vi "ROI entry-Index Zplane position.vi"(8 "error in (no error)":errorcluster, 11 "Init?":bool) -> (0 "error out":errorcluster, 3 "Z-plane selector (index)":i32)   [LabVIEW 2013]
uses:
  ROI Entry screen/Globals/gl_ROI Entry UI globals.vi
panel:
  out "Zplane position":dbl
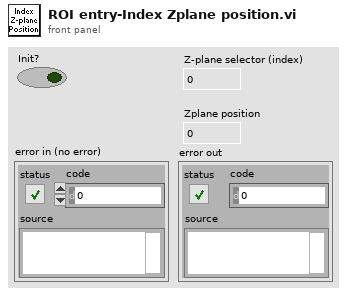
[diagram p1: front panel]
types:
  T1 = typedef "ROI entry screen ctrl refs cluster.ctl" = cluster{"Done button":refnum<vi>, "Imaging button":refnum<vi>, "Acquisition button":refnum<vi>, "POI dwell time (us)":refnum<vi>, "Scan dwell time per pixel (us)":refnum<vi>, "# of planes":refnum<vi>, "Zoom":refnum<vi>, "Equal size":refnum<vi>, "Channel":refnum<vi>, "Image Display":refnum<vi>, "Z-Plane Selector":refnum<vi>, "Number of lines left":refnum<vi>, "Z-stack folder path":refnum<vi>, "POI Density":refnum<vi>, "Arb Plane Entry":refnum<vi>, "Whole plane":refnum<vi>, "Clear Last":refnum<vi>, "Clear All":refnum<vi>, "Trial Length (sec)":refnum<vi>, "Palette Type":refnum<vi>, "Intensity slider":refnum<vi>, "# POI":refnum<vi>, "Max Z Proj":refnum<vi>, "Zplane ind":refnum<vi>, "Wavelength (nm)":refnum<vi>, "Number of Trials":refnum<vi>, "Funct stim.trig.enable":refnum<vi>, "Funct stim.trig.delay (s)":refnum<vi>, "Line Mode":refnum<vi>, "Step size (µm)":refnum<vi>, "ROI move mode":refnum<vi>, "Cool-down time (s)":refnum<vi>, "Enable cool-down time":refnum<vi>, "Motor Z ind. (um)":refnum<vi>, "AOL Z ind. (um)":refnum<vi>}
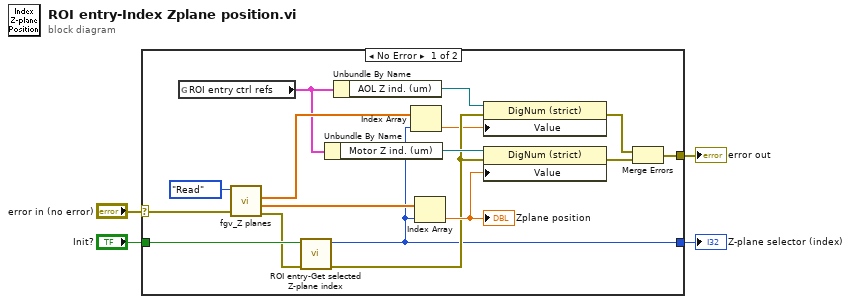
[diagram p0: block diagram]
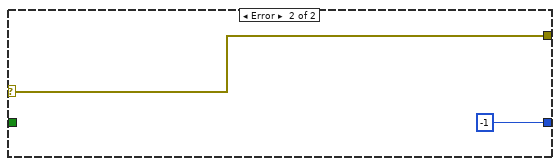
[diagram p2: hidden frame]
diagram:
  n1 = case shown="No Error" "error in (no error)" {
    selector: "error in (no error)" -> [w15 w22]
    tunnel: "Init?" -> [w20 _]
    tunnel: [w9 -1 ("Z-plane selector (index)")] -> w3
    tunnel: [w10 w22] -> w1
    frame No Error {
      n2 = global read "gl_ROI Entry UI globals.vi" "ROI entry ctrl refs"() -> (w5:T1)
      n3 = call "fgv_Z planes.vi"("error in (no error)"=w15, "Function"=enum16{"Intialize", "Write", "Read", "Clear"}."Read") -> ("error out"=w16:errorcluster, "Motor Z planes"=w17:dbl[], "AOL Z Planes"=w7:dbl[])  [unwired: 7 in]
      n4 = call "ROI entry-Get selected Z-plane index.vi"("error in (no error)"=w16, "Initialisation"=w20) -> ("error out"=w13:errorcluster, "Z-plane selector (index)"=w9:i32)  [unwired: 8 in]
      n5 = Unbundle By Name(w5) -> ("Motor Z ind. (um)"=w19:refnum<vi>)
      n6 = Unbundle By Name(w5) -> ("AOL Z ind. (um)"=w6:refnum<vi>)
      n7 = Index Array(array=w7, index=w9) -> (element=w8:dbl)
      n8 = Index Array(array=w17, index=w9) -> (element=w14:dbl)
      "Zplane position" <- w14
      n9 = property on="Property Node" class="DigNum (strict)"(reference=w6, error in=w13, "Value"=w8) -> (error out=w12:errorcluster)  [unwired: 1 out]
      n10 = property on="Property Node" class="DigNum (strict)"(reference=w19, error in=w13, "Value"=w14) -> (error out=w11:errorcluster)  [unwired: 1 out]
      n11 = Merge Errors(w12, w11) -> (w10:errorcluster)
    }
    frame Error {
    }
  }
  "Z-plane selector (index)" <- w3
  "error out" <- w1
